vi "AO Update.vi"(8 "error in":errorcluster, 9 "AO Timing":T2={"samples per channel"=1000, "sample mode"=10178, "Sampling Rate"=1000.0} {"sample mode" items=["Finite Samples"=10178, "Continuous Samples"=10123, "Hardware Timed Single Point"=12522]}, 10 "Interupt Q":refnum<queue>, 11 "Configuration Data":T1[](array[typedef])) -> (0 "error out":errorcluster, 1 "Stop":bool, 2 "Data To Generate":waveform(dbl)[](array[waveform]), 3 "Configuration Data":T1[](array[typedef]))   [LabVIEW 2024]
doc: "All Rights Reserved © 2017 SyncSols"
uses:
  TCP Engine/Controls/TCP Engine I&O  Interupt Cluster.ctl
  Controls/AO Channel Configuration Cluster.ctl
  Controls/AO Timing Cluster.ctl
  Controls/AO 1D DBL ArrayCluster.ctl
  Controls/AO 1D DBL Interface Data Cluster.ctl
  Controls/AO DBL Data Cluster.ctl
  TCP Engine/TCP Engine.lvlib
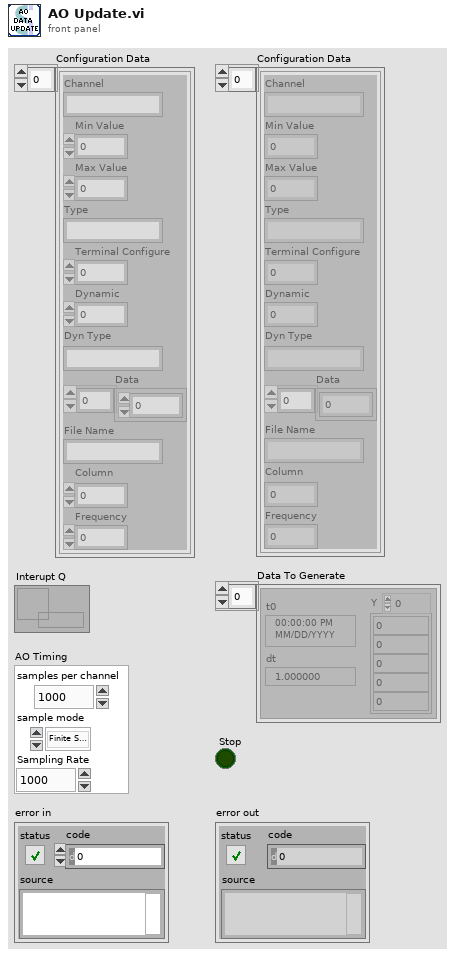
[diagram p1: front panel]
types:
  T1 = typedef "AO Channel Configuration Cluster.ctl" = cluster{"Channel":string, "Min Value":dbl, "Max Value":dbl, "Type":string, "Terminal Configure":u16, "Dynamic":u8, "Dyn Type":string, "Data":dbl[], "File Name":string, "Column":i32, "Frequency":dbl}
  T2 = typedef "AO Timing Cluster.ctl" = cluster{"samples per channel":i32, "sample mode":i32, "Sampling Rate":dbl}
  T3 = typedef "AO 1D DBL ArrayCluster.ctl" = cluster{"Interface":string, "Interface Data":T4}
  T4 = typedef "AO 1D DBL Interface Data Cluster.ctl" = cluster{"Command":string, "SubCmd":string, "Data":T5[]}
  T5 = typedef "AO DBL Data Cluster.ctl" = cluster{"Channel":string, "Data":dbl}
  T6 = typedef "TCP Engine.lvlib/TCP Engine I&O  Interupt Cluster.ctl" = cluster{" Stop":bool, "JSON Variant":variant}
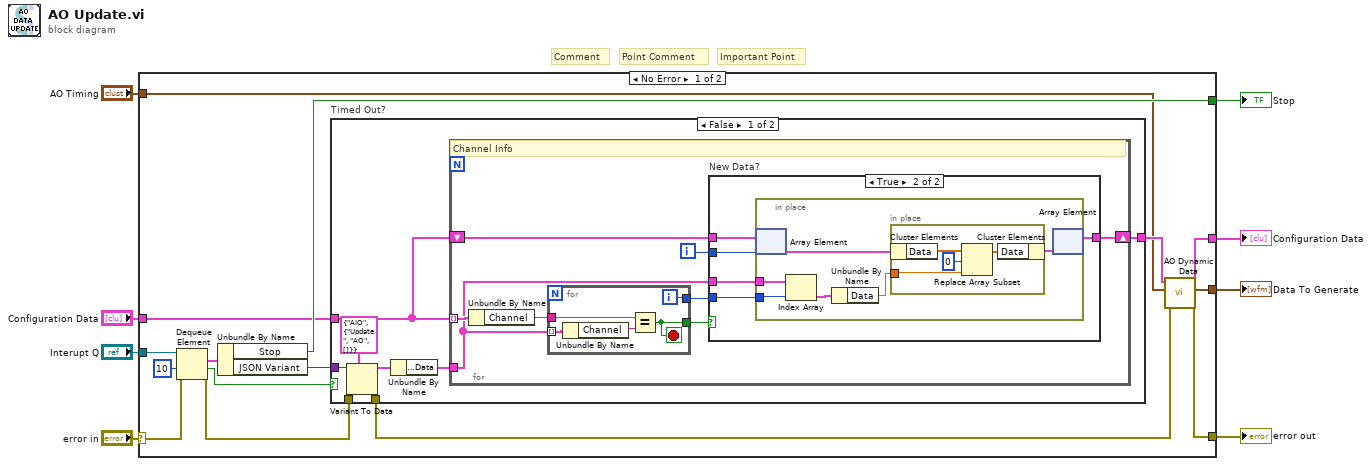
[diagram p0: block diagram]
diagram:
  # "Important Point"
  # "Point Comment"
  # "Comment"
  n1 = case shown="No Error" "error in" {
    selector: "error in" -> [w20 w64]
    tunnel: [w9 w64] -> w8
    tunnel: "Interupt Q" -> [w21 _]
    tunnel: [w16 _] -> w5
    tunnel: "Configuration Data" -> [w15 w63]
    tunnel: "AO Timing" -> [w13 _]
    tunnel: [w12 w63] -> w1
    tunnel: [w11 _] -> w2
    frame No Error {
      n2 = Dequeue Element(queue=w21, timeout in ms (-1)=10, error in (no error)=w20) -> (element=w22:T6, timed out?=w19:bool, error out=w18:errorcluster)  [unwired: 1 out]
      n3 = Unbundle By Name(w22) -> ("Stop"=w16:bool, "JSON Variant"=w17:variant)
      n4 = case "Timed Out?" shown="False" w19 {
        tunnel: w18 -> [w31 w62]
        tunnel: [w30 w62] -> w10
        tunnel: w17 -> [w29 _]
        tunnel: w15 -> [w25 w61]
        tunnel: [w24 w61] -> w14
        frame False {
          n5 = Variant To Data(error in=w31, type=T3 {"Interface"="AIO", "Interface Data"={"Command"="Update", "SubCmd"="AO", "Data"=[]}}, Variant=w29) -> (data=w28:T3, error out=w30:errorcluster)
          n6 = Unbundle By Name(w28) -> ("Interface Data.Data"=w26:T5[])
          n7 = for {
            tunnel: w25 -> [w39] mode=indexing
            tunnel: w26 -> [w36]
            shift-right: [w32] -> w24
            shift-left: w25 -> [w35]
            i -> [w33]
            # "Channel Info"
            n8 = Unbundle By Name(w39) -> ("Channel"=w38:string)
            n9 = for {
              tunnel: w38 -> [w58]
              tunnel: w36 -> [w60] mode=indexing
              tunnel: [w57] -> w37
              tunnel: [w56] -> w34
              i -> [w56]
              stop <- w57 stop-if-true
              n10 = Unbundle By Name(w60) -> ("Channel"=w59:string)
              n11 = Equal?(x=w58, y=w59) -> (x = y?=w57:bool)
            }
            n12 = case "New Data?" shown="True" w37 {
              tunnel: w36 -> [_ w45]
              tunnel: w35 -> [w40 w43]
              tunnel: w34 -> [_ w44]
              tunnel: w33 -> [_ w42]
              tunnel: [w40 w41] -> w32
              frame False {
              }
              frame True {
                n13 = in-place {
                  in-place-border: w45 -> [w51]
                  in-place-border: w44 -> [w50]
                  n14 = in-place-array #1(w43, w42) -> (w47:T1)
                  n15 = Index Array(array=w51, index=w50) -> (element=w49:T5)
                  n16 = Unbundle By Name(w49) -> ("Data"=w48:dbl)
                  n17 = in-place {
                    in-place-border: w48 -> [w55]
                    n18 = in-place-cluster #2(w47) -> ("Data"=w52:dbl[])
                    n19 = Replace Array Subset(array=w52, new element=w55, index=0) -> (w54:dbl[])
                    n20 = in-place-cluster #2("Data"=w54) -> (w46:T1)
                  }
                  n21 = in-place-array #1(w46) -> (w41:T1[])  [unwired: 1 out]
                }
              }
            }
          }
        }
        frame True {
        }
      }
      n22 = call "AO Dynamic Data.vi"("error in"=w10, "AO Timing"=w13, "Configuration Data"=w14) -> ("error out"=w9:errorcluster, "Data To Generate"=w11:waveform(dbl)[], "Configuration Data Out"=w12:T1[])  [unwired: 6 in]
    }
    frame Error {
    }
  }
  "error out" <- w8
  "Stop" <- w5
  "Data To Generate" <- w2
  "Configuration Data" <- w1
